vi "Set Variant Property.vi"(6 "Control Ref Queue":T1, 8 "error in (no error)":errorcluster, 10 "Property In":variant, 11 "3D Pie.lvclass in":refnum<class "3D Pie.lvclass">) -> (0 "error out":errorcluster, 3 "3D Pie.lvclass":refnum<class "3D Pie.lvclass">)   [LabVIEW 2020, in "3D Pie.lvclass"]
uses:
  <vilib>/Math Plots/3D Math Plots/3D Pie/3D Pie/3D Pie.lvclass
  <vilib>/Math Plots/3D Math Plots/3D Pie/3D Pie/Typedef/3D Pie Property Array.ctl
  <vilib>/Math Plots/3D Math Plots/3D Pie/3D Pie/Typedef/3D Pie Property.ctl
  <vilib>/Math Plots/3D Math Plots/3D Plot/3D Plot/Typedef/Line Type.ctl
  <vilib>/Math Plots/3D Math Plots/3D Plot/Action String/3DMathPlot Ctrl Act Queue.ctl
  <vilib>/Math Plots/3D Math Plots/3D Plot/Action String/3DMathPlot Ctrl Act Cluster.ctl
  <vilib>/Math Plots/3D Math Plots/3D Plot/Action String/3DMathPlot State Class.ctl
  <vilib>/Math Plots/3D Math Plots/3D Pie/3D Pie/3D Pie.lvclass/3D Pie.ctl
  <vilib>/Math Plots/3D Math Plots/3D Plot/3D Plot/3D Plot.lvclass
panel:
  in  "3D Pie Property Array":T2
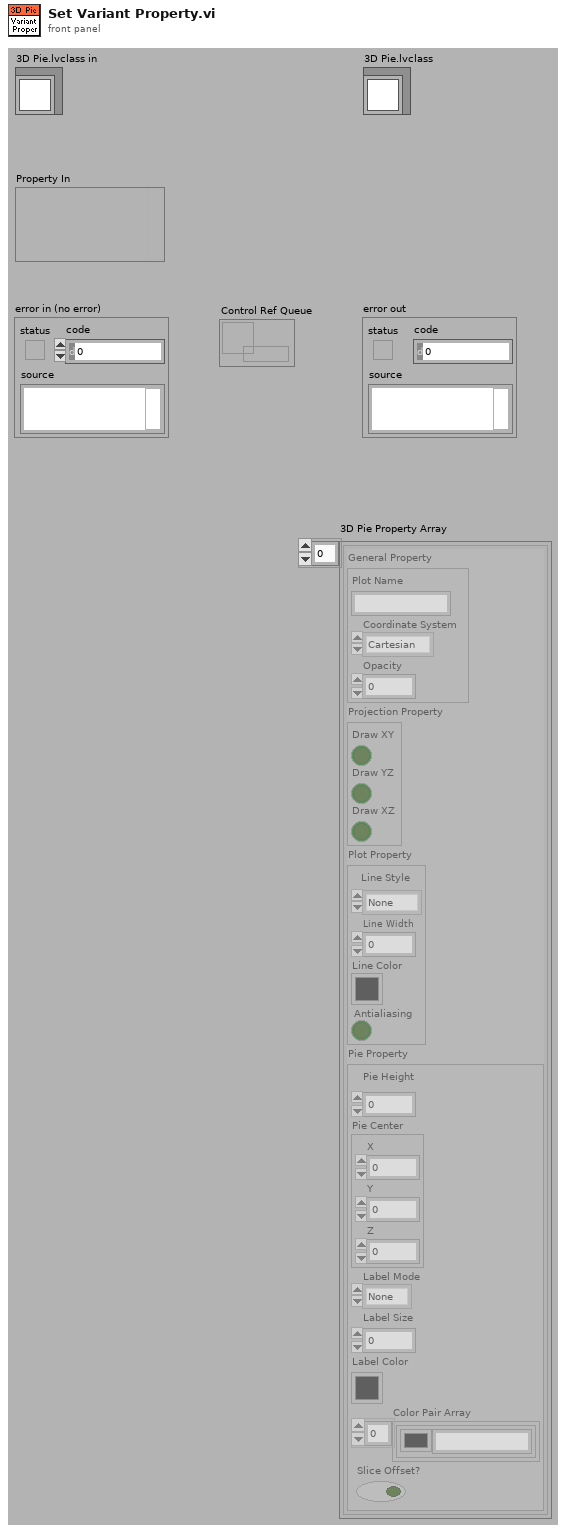
[diagram p1: front panel]
types:
  T1 = typedef "3DMathPlot Ctrl Act Queue.ctl" = refnum<queue>
  T2 = typedef "3D Pie.lvclass/3D Pie Property Array.ctl" = T3[]
  T3 = typedef "3D Pie.lvclass/3D Pie Property.ctl" = cluster{"General Property":cluster{"Plot Name":string, "Coordinate System":enum16{"Cartesian", "Cylindrical", "Spherical"}, "Opacity":sgl}, "Projection Property":cluster{"Draw XY":bool, "Draw YZ":bool, "Draw XZ":bool}, "Plot Property":cluster{"Line Style":T4, "Line Width":sgl, "Line Color":u32, "Antialiasing":bool}, "Pie Property":cluster{"Pie Height":sgl, "Pie Center":cluster{"X":sgl, "Y":sgl, "Z":sgl}, "Label Mode":enum16{"None", "Show Percentage", "Show String"}, "Label Size":u16, "Label Color":u32, "Color Pair Array":cluster{"Color":u32, "String":string}[], "Slice Offset?":bool}}
  T4 = typedef "3D Plot.lvclass/Line Type.ctl" = enum16{"None", "Solid", "Dash", "Dot", "Dash Dot"}
  T5 = typedef "3DMathPlot State Class.ctl" = enum16{"Update All Objects (Undo)", "Update Light Object Only", "Update Axis Object Only", "Update Plot Object Only", "Update Cursor Object Only", "Update Axis Plot Cursor Objects", "No Update"}
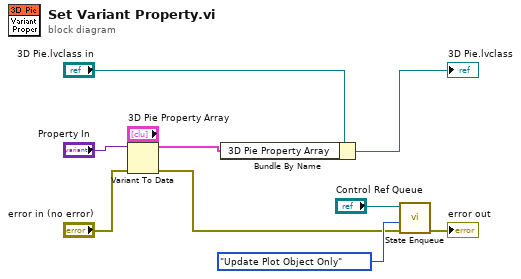
[diagram p0: block diagram]
diagram:
  n1 = Variant To Data(error in="error in (no error)", type="3D Pie Property Array", Variant="Property In") -> (data=w10:T2, error out=w2:errorcluster)
  n2 = Bundle By Name(cluster="3D Pie.lvclass in", "3D Pie Property Array"=w10) -> (→"3D Pie.lvclass":refnum<class "3D Pie.lvclass">)
  n3 = call <vilib>:"State Enqueue.vi"("error in (no error)"=w2, "Display State Change Class"=3DMathPlot_State_Class."Update Plot Object Only", "Control Ref Queue"="Control Ref Queue") -> ("error out"=→"error out":errorcluster)  [unwired: 8 out]
